vi "ResearcgStandingFrame-V1.1.vi"() -> ()   [LabVIEW 2012]
doc: "Use this template to build a simple state machine design pattern. Each state executes code and determines which state to transition to."
uses:
  controls/State.ctl
panel:
  out "appended array":dbl[](array[numeric])
  out "Scalar":dbl
  out "text":string
  out "substring":string
  in  "Tab Control":T1(tab)
  out "Center Mass Left Force Plate":cluster{dbl[], dbl[]}(graph)={[-7.494780644696312], [-1.1979086821741642]}
  in  "Begin":bool
  in  "stop":bool
  out "Newton Force Readings File Path":path=path "C:/Documents and Settings/z00323/My Documents/Standing Frame/test data/StandingFrameTEST39.dat"
  in  "Newtons":bool
  out "Voltage Readings File Path":path=path "C:/Documents and Settings/z00323/My Documents/Standing Frame/test data/StandingFrameTEST39.dat"
  out "R-FP-Z":dbl
  out "R-FP-Y":dbl
  out "R-FP-X":dbl
  out "R-LC-Z":dbl
  out "R-LC-Y":dbl
  out "R-LC-X":dbl
  out "L-LC-Z":dbl
  out "L-LC-Y":dbl
  out "L-LC-X":dbl
  out "L-FP-X":dbl
  out "L-FP-Y":dbl
  out "L-FP-Z":dbl
  out "String":string caption="Display Unit"
  out "Left Force Plate Z":dbl(slide)=0.43558763460600747 scale=0.0..250.0
  out "Right Force Plate Z":dbl(slide)=0.868584773555102 scale=0.0..250.0
  out "Center Mass Right Force Plate":cluster{dbl[], dbl[]}(graph)
  out "Right Load Cell":cluster{dbl[], dbl[]}(graph)={[0.0, -0.0006862149399022939, 0.0, 0.0], [0.0, 0.005798023167495851, 0.0, 0.0]}
  out "Right Load Cell Z":dbl(slide)=-0.000301685706272135 scale=-50.0..250.0
  out "Left Load Cell Z":dbl(slide)=-0.004073381073294343 scale=-50.0..250.0
  out "Left Load Cell":cluster{dbl[], dbl[]}(graph)={[0.0, -0.0004854170425343219, 0.0, 0.0], [0.0, -0.002818533162237429, 0.0, 0.0]}
  out "Amplitude Unit":string
  out "Right Force PLate Z":dbl(graph)
  out "Left Force Plate Z":dbl(graph)
  out "Right Load Cell Z":dbl(graph)
  out "Right Load Cell Y":dbl(graph)
  out "Right Load Cell X":dbl(graph)
  out "Left Load Cell Z":dbl(graph)
  out "Left Load Cell Y":dbl(graph)
  out "Left Load Cell X":dbl(graph)
  out "Amplitude Unit":string
  in  "Loading- Clibration File Path":path
  in  "Save Calibration Results":bool
  in  "Load Previous Calibration Results":bool
  out "Saving- Clibration File Path":path
  out "Baseline Out":dbl[](array[numeric])
  out "Voltages":dbl[](array[numeric])
  in  "New Calibration":bool
  # "Left Load Cell X\n\nLeft Load Cell Y\n\n\nLeft Load Cell Z\n\nRight Load Cell X\n\n\nRight Load Cell Y\n\nRight Load Cell Z\n\n\nLeft Force Plate X1\n\nLeft Force Plate X2\n\n\nLeft Force Plate Y1\n\nLeft Force PLate Y2\n\n\nLeft Force Plate Z1\n\nLeft Force Plate Z2\n\n\nLeft Force Plate Z3\n\nLeft Force Plate Z4\n\n\nRight Force Plate X1\n\nRight Force Plate X2\n\n\nRight Force Plate Y1\n\nRight Force PLate Y2\n\n\nRight Force Plate Z1\n\nRight Force Plate Z2\n\n\nRight Force Plate Z3\n\nRight Force Plate Z4"
  # "DAQ Board Connections"
  # "LX\nLY\nLZ\nRX\nRY\nRZ\nLFX12\nLFX34\nLFY14\nLFY23\nLFZ1\nLFZ2\nLFZ3\nLFZ4\nRFX12\nRFX34\nRFY14\nRFY23\nRFZ1\nRFZ2\nRFZ3\nRFZ4"
  # "32\n33\n34\n35\n36\n37\n0\n1\n2\n3\n4\n5\n6\n7\n16\n17\n18\n19\n20\n21\n22\n23"
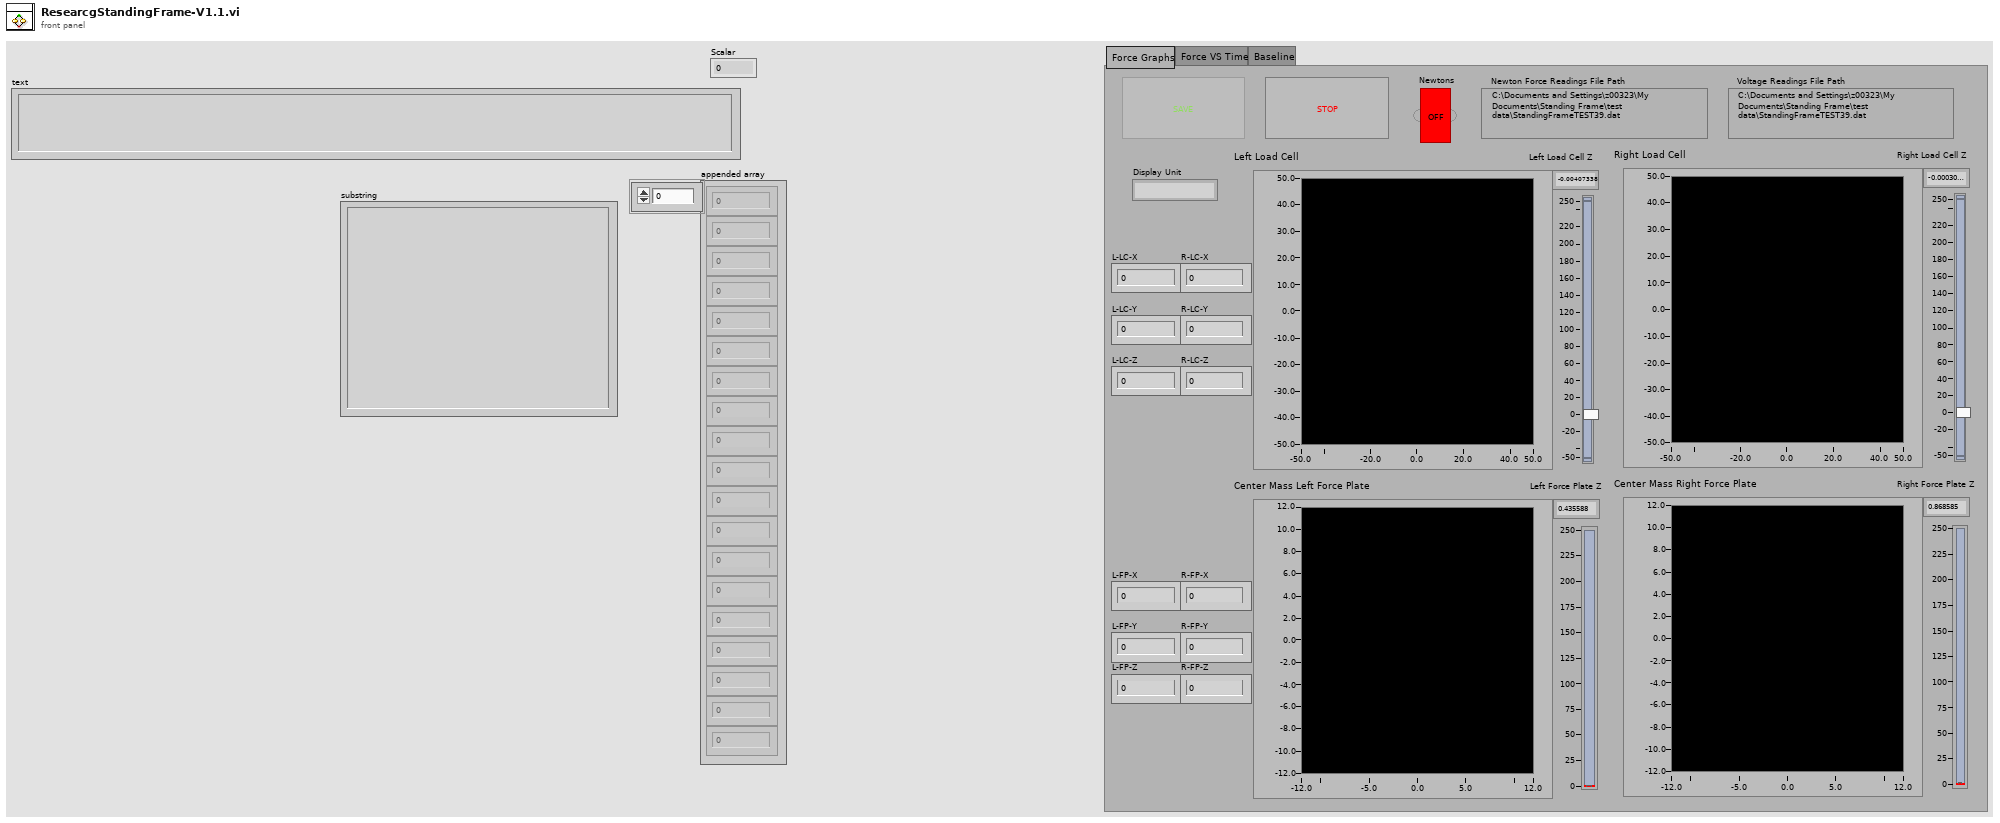
[diagram p1: front panel]
types:
  T1 = enum32{"Force Graphs", "Force VS Time", "Baseline"}
  T2 = typedef "State.ctl" = enum16{"Initialize", "Save", "Main", "Stop"}
  T3 = enum16{"open", "replace", "create", "open or create", "replace or create", "replace or create with confirmation"}
  T4 = enum8{"Enabled", "Disabled", "Disabled and Grayed Out"}
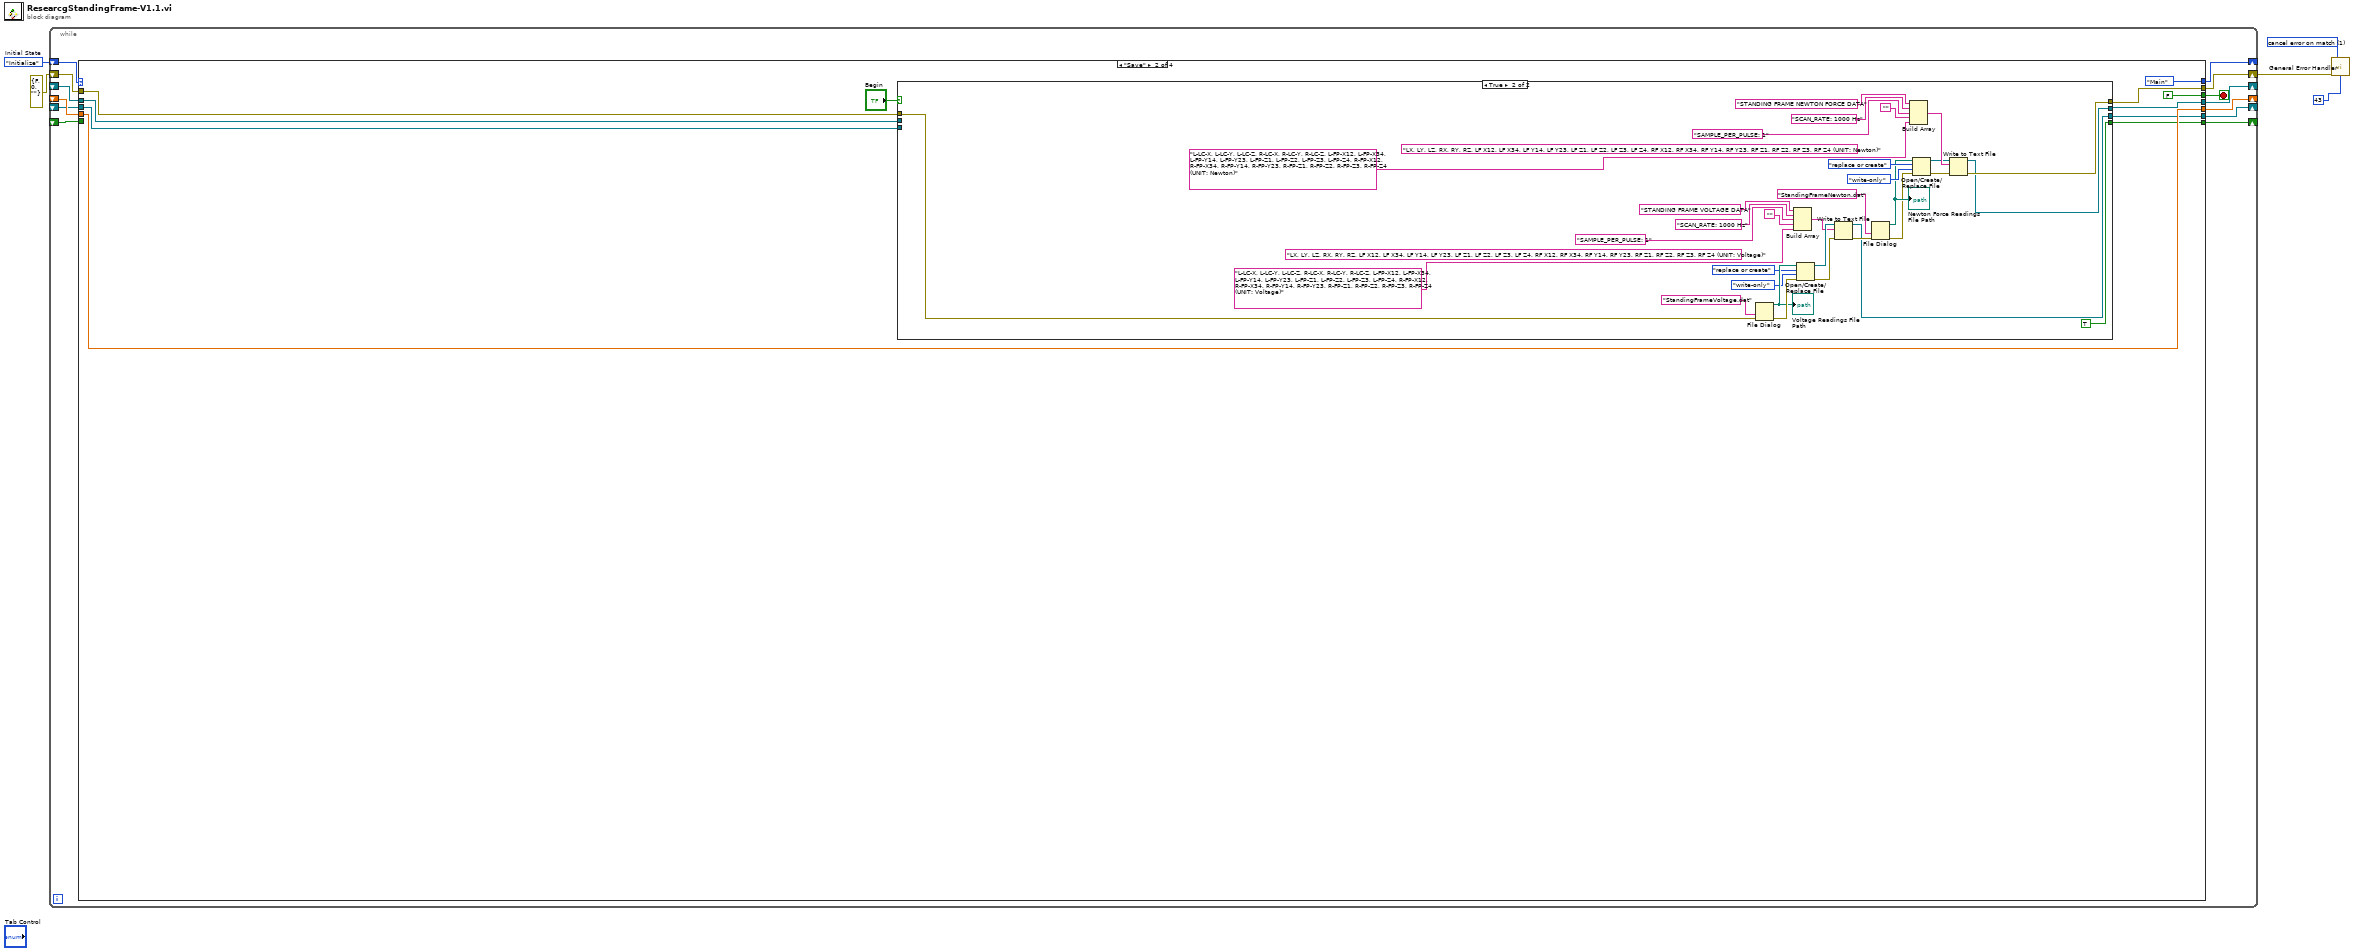
[diagram p0: block diagram]
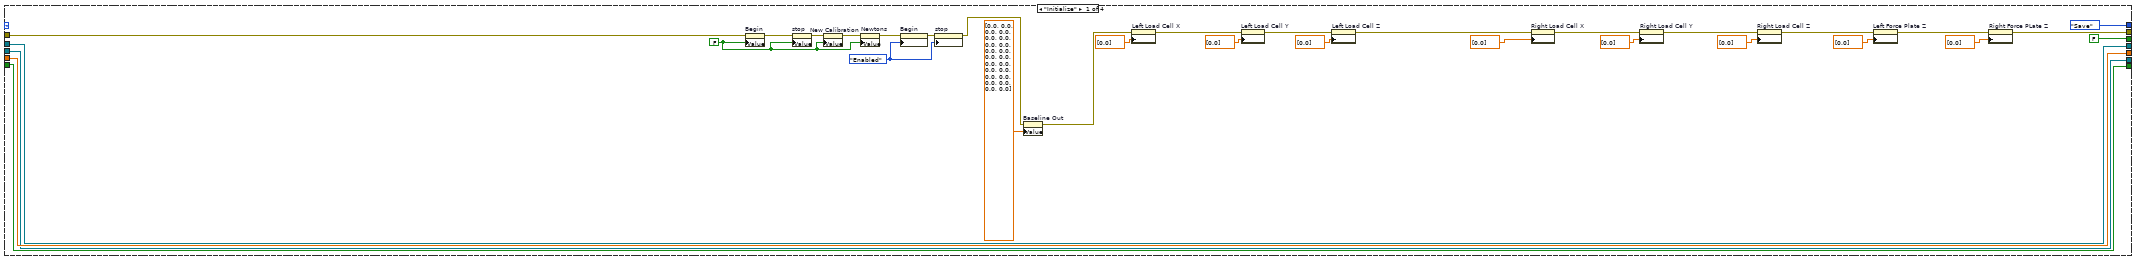
[diagram p2: hidden frame]
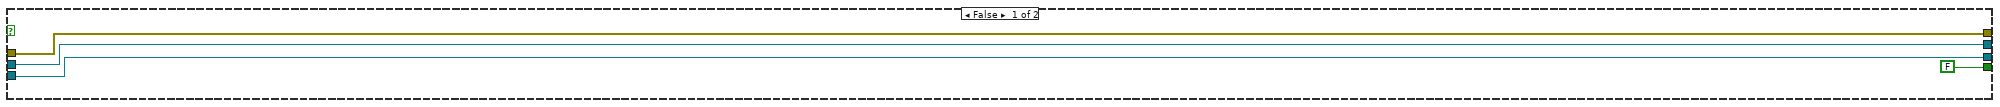
[diagram p3: hidden frame]
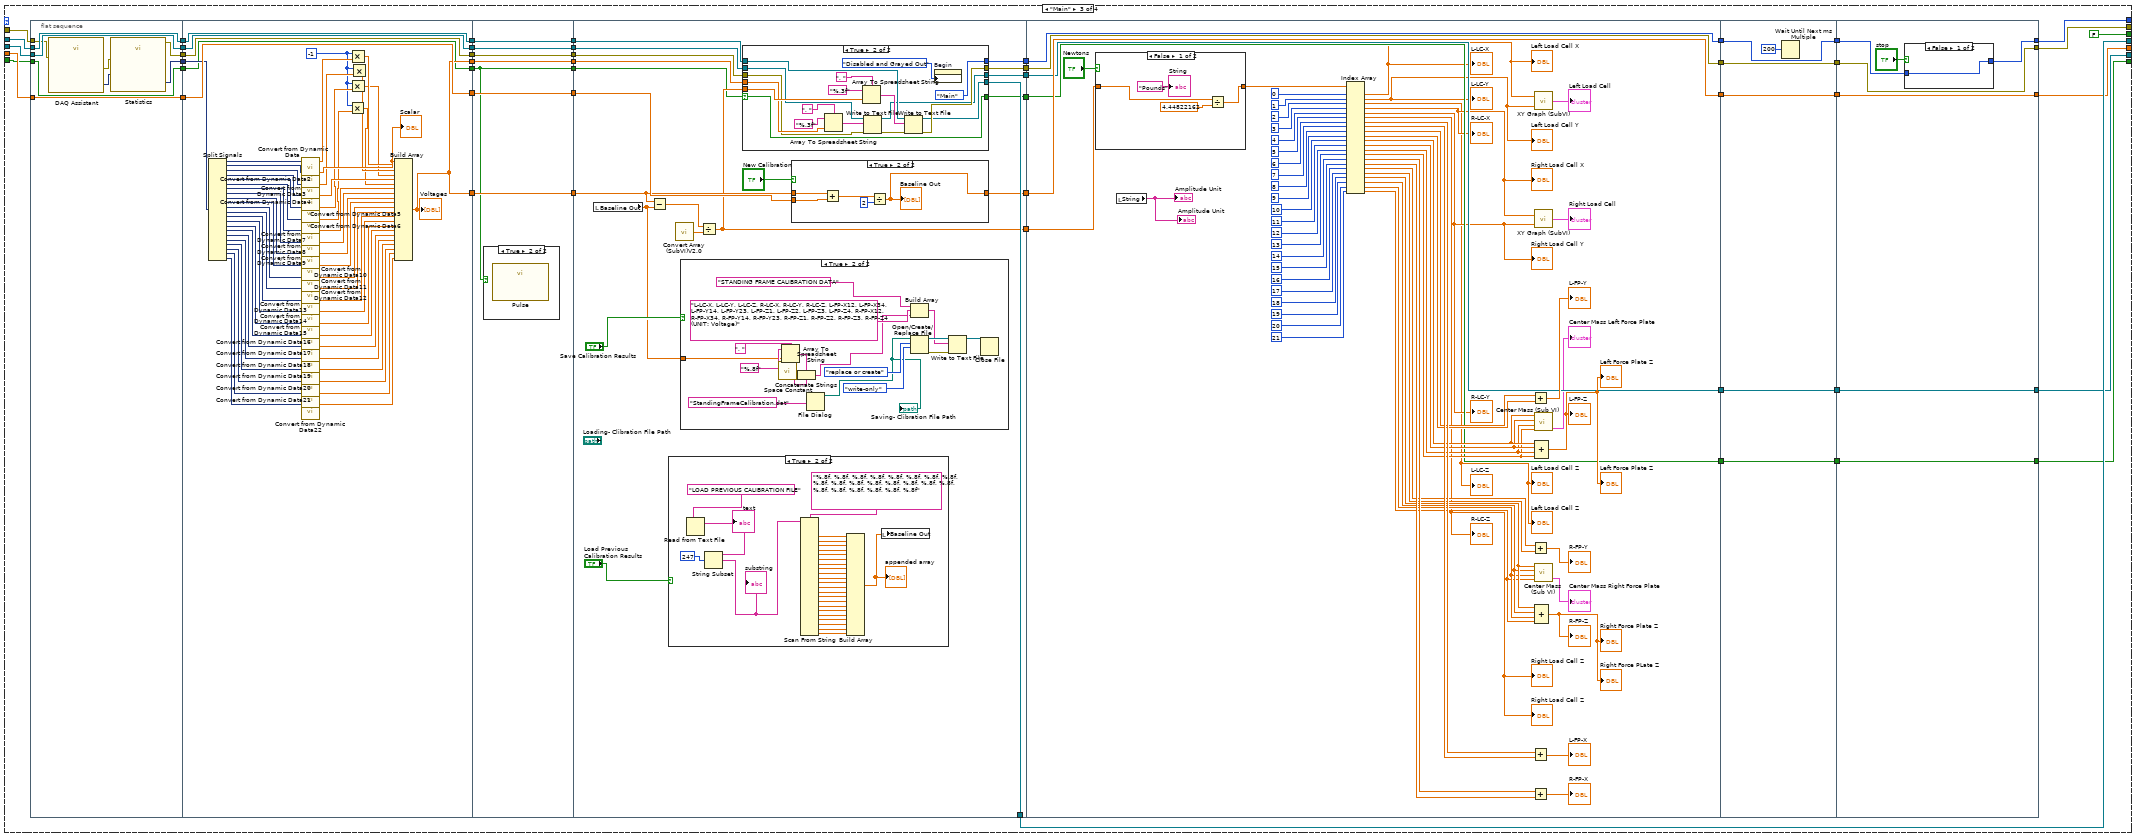
[diagram p4: hidden frame]
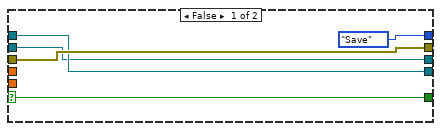
[diagram p8: hidden frame]
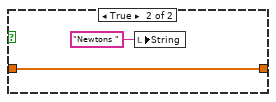
[diagram p10: hidden frame]
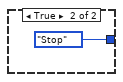
[diagram p11: hidden frame]
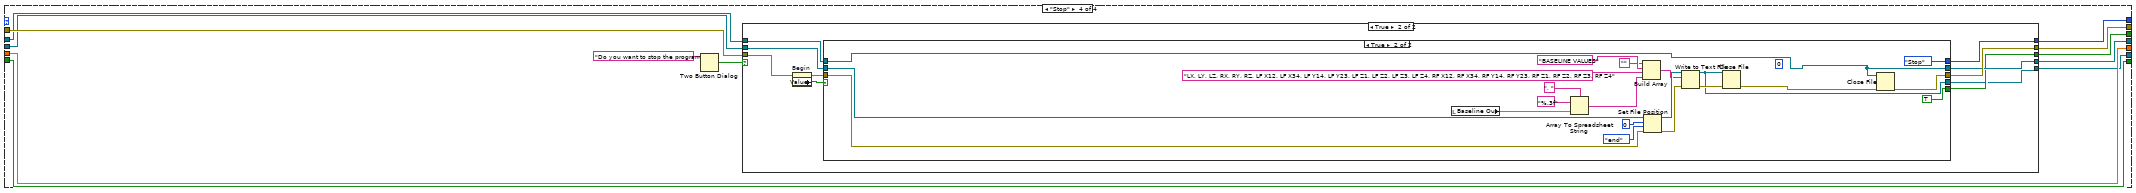
[diagram p12: hidden frame]
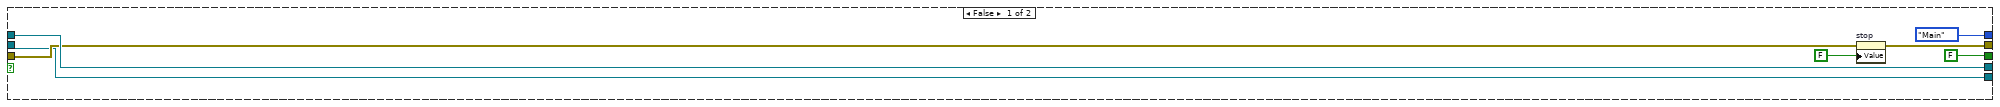
[diagram p13: hidden frame]
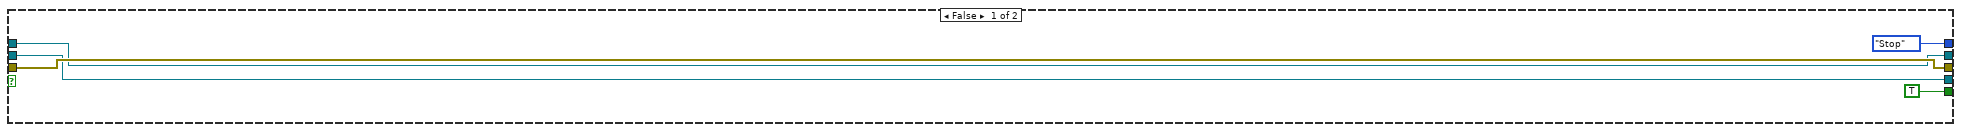
[diagram p14: hidden frame]
diagram:
  w1 = 1 items=["no exception", "cancel error on match", "set error on match"] ("[exception action] (none:0)")
  w5 = State."Initialize"  # Initial State
  n1 = while {
    shift-right: [w17] -> _
    shift-left: w5 -> [w18]
    shift-right: [w12] -> w3
    shift-left: errorcluster {"status"=FALSE, "code"=0, "source"=""} ("error out") -> [w16]
    shift-right: [w14] -> _
    shift-left: _ -> [w13]
    shift-right: [w10] -> _
    shift-left: _ -> [w11]
    shift-right: [w9] -> _
    shift-left: _ -> [w8]
    shift-right: [w7] -> _
    shift-left: _ -> [w6]
    stop <- w15 stop-if-true
    n2 = case shown="\"Save\"" w18 {
      tunnel: [State."Save" ("Next State") State."Main" ("Next State") w144 w405] -> w17
      tunnel: [FALSE ("T button?") FALSE FALSE ("T button?") w404] -> w15
      tunnel: w16 -> [w45 w60 w146 w403]
      tunnel: [w49 w59 w139 w400] -> w14
      tunnel: w13 -> [w49 w56 w145 w401]
      tunnel: [w21 w58 w131 w402] -> w12
      tunnel: w11 -> [w44 w55 w129 w399]
      tunnel: [w44 w55 w125 w399] -> w10
      tunnel: [w41 w52 w124 w398] -> w9
      tunnel: w8 -> [w41 w54 w119 w397]
      tunnel: [w19 w53 w116 w396] -> w7
      tunnel: w6 -> [w19 _ w117 w396]
      frame "Initialize" {
        w38 = FALSE ("Begin")
        w48 = T4."Enabled" ("Disabled")
        n3 = property on="Begin" class="Bool (strict)"(error in=w45, "Value"=w38) -> (error out=w47:errorcluster)  [unwired: 1 in, 1 out]
        n4 = property on="stop" class="Bool (strict)"(error in=w47, "Value"=w38) -> (error out=w43:errorcluster)  [unwired: 1 in, 1 out]
        n5 = property on="New Calibration" class="Bool (strict)"(error in=w43, "Value"=w38) -> (error out=w40:errorcluster)  [unwired: 1 in, 1 out]
        n6 = property on="Newtons" class="Bool (strict)"(error in=w40, "Value"=w38) -> (error out=w39:errorcluster)  [unwired: 1 in, 1 out]
        n7 = property on="Begin" class="Bool (strict)"(error in=w39, "DisabledEnum"=w48) -> (error out=w46:errorcluster)  [unwired: 1 in, 1 out]
        n8 = property on="stop" class="Bool (strict)"(error in=w46, "DisabledEnum"=w48) -> (error out=w20:errorcluster)  [unwired: 1 in, 1 out]
        n9 = property on="Baseline Out" class="Arr (strict)"(error in=w20, "Value"=dbl[] [0.0, 0.0, 0.0, 0.0, 0.0, 0.0, 0.0, 0.0, 0.0, 0.0, 0.0, 0.0, 0.0, 0.0, 0.0, 0.0, 0.0, 0.0, 0.0, 0.0, 0.0, 0.0] ("Baseline Out")) -> (error out=w29:errorcluster)  [unwired: 1 in, 1 out]
        n10 = property on="Left Load Cell X" class="WFChart (strict)"(error in=w29, "History Data"=dbl[] [0.0]) -> (error out=w28:errorcluster)  [unwired: 1 in, 1 out]
        n11 = property on="Left Load Cell Y" class="WFChart (strict)"(error in=w28, "History Data"=dbl[] [0.0]) -> (error out=w27:errorcluster)  [unwired: 1 in, 1 out]
        n12 = property on="Left Load Cell Z" class="WFChart (strict)"(error in=w27, "History Data"=dbl[] [0.0]) -> (error out=w26:errorcluster)  [unwired: 1 in, 1 out]
        n13 = property on="Right Load Cell X" class="WFChart (strict)"(error in=w26, "History Data"=dbl[] [0.0]) -> (error out=w25:errorcluster)  [unwired: 1 in, 1 out]
        n14 = property on="Right Load Cell Y" class="WFChart (strict)"(error in=w25, "History Data"=dbl[] [0.0]) -> (error out=w24:errorcluster)  [unwired: 1 in, 1 out]
        n15 = property on="Right Load Cell Z" class="WFChart (strict)"(error in=w24, "History Data"=dbl[] [0.0]) -> (error out=w23:errorcluster)  [unwired: 1 in, 1 out]
        n16 = property on="Left Force Plate Z" class="WFChart (strict)"(error in=w23, "History Data"=dbl[] [0.0]) -> (error out=w22:errorcluster)  [unwired: 1 in, 1 out]
        n17 = property on="Right Force PLate Z" class="WFChart (strict)"(error in=w22, "History Data"=dbl[] [0.0]) -> (error out=w21:errorcluster)  [unwired: 1 in, 1 out]
      }
      frame "Save" {
        n18 = case shown="True" "Begin" {
          tunnel: w60 -> [w66 w78]
          tunnel: [w65 w92] -> w59
          tunnel: [w66 w94] -> w58
          tunnel: w56 -> [w65 _]
          tunnel: [w64 w76] -> w52
          tunnel: w54 -> [w64 _]
          tunnel: [FALSE TRUE] -> w53
          frame False {
          }
          frame True {
            (unwired) "LX, LY, LZ, RX, RY, RZ, LF X12, LF X34, LF Y14, LF Y23, LF Z1, LF Z2, LF Z3, LF Z4, RF X12, RF X34, RF Y14, RF Y23, RF Z1, RF Z2, RF Z3, RF Z4 (UNIT: Voltage)"
            (unwired) "LX, LY, LZ, RX, RY, RZ, LF X12, LF X34, LF Y14, LF Y23, LF Z1, LF Z2, LF Z3, LF Z4, RF X12, RF X34, RF Y14, RF Y23, RF Z1, RF Z2, RF Z3, RF Z4 (UNIT: Newton)"
            n19 = File Dialog(8:w78, 9:"StandingFrameVoltage.dat" ("default name")) -> (0:w86:errorcluster, 3:w84:path)  [unwired: 1 in, 6 out]
            "Voltage Readings File Path" <- w84
            n20 = Build Array("STANDING FRAME VOLTAGE DATA", "SCAN_RATE: 1000 Hz", "SAMPLE_PER_PULSE: 1", "", "L-LC-X, L-LC-Y, L-LC-Z, R-LC-X, R-LC-Y, R-LC-Z, L-FP-X12, L-FP-X34, L-FP-Y14, L-FP-Y23, L-FP-Z1, L-FP-Z2, L-FP-Z3, L-FP-Z4, R-FP-X12, R-FP-X34, R-FP-Y14, R-FP-Y23, R-FP-Z1, R-FP-Z2, R-FP-Z3, R-FP-Z4 (UNIT: Voltage)") -> (w82:string[])
            n21 = Open/Create/Replace File(file path (use dialog)=w84, error in=w86, operation (0:open)=T3."replace or create", access (0:read/write)=enum16{"read/write", "read-only", "write-only"}."write-only") -> (refnum out=w83:refnum<file>, error out=w87:errorcluster)  [unwired: 3 out]
            n22 = Write to Text File(file (use dialog)=w83, text=w82, error in=w87) -> (refnum out=w76:refnum<file>, error out=w77:errorcluster)  [unwired: 1 in, 1 out]
            n23 = File Dialog(8:w77, 9:"StandingFrameNewton.dat" ("default name")) -> (0:w89:errorcluster, 3:w91:path)  [unwired: 1 in, 6 out]
            "Newton Force Readings File Path" <- w91
            n24 = Build Array("STANDING FRAME NEWTON FORCE DATA", "SCAN_RATE: 1000 Hz", "SAMPLE_PER_PULSE: 1", "", "L-LC-X, L-LC-Y, L-LC-Z, R-LC-X, R-LC-Y, R-LC-Z, L-FP-X12, L-FP-X34, L-FP-Y14, L-FP-Y23, L-FP-Z1, L-FP-Z2, L-FP-Z3, L-FP-Z4, R-FP-X12, R-FP-X34, R-FP-Y14, R-FP-Y23, R-FP-Z1, R-FP-Z2, R-FP-Z3, R-FP-Z4 (UNIT: Newton)") -> (w95:string[])
            n25 = Open/Create/Replace File(file path (use dialog)=w91, error in=w89, operation (0:open)=T3."replace or create", access (0:read/write)=enum16{"read/write", "read-only", "write-only"}."write-only") -> (refnum out=w93:refnum<file>, error out=w88:errorcluster)  [unwired: 3 out]
            n26 = Write to Text File(file (use dialog)=w93, text=w95, error in=w88) -> (refnum out=w92:refnum<file>, error out=w94:errorcluster)  [unwired: 1 in, 1 out]
          }
        }
      }
      frame "Main" {
        n27 = flat-sequence {
          tunnel: w146 -> [w150]
          tunnel: w145 -> [w153]
          tunnel: [w155] -> w142
          tunnel: [w154] -> w141
          tunnel: [w153] -> w140
          tunnel: [w152] -> w130
          tunnel: w129 -> [w152]
          tunnel: [w151] -> w120
          tunnel: w119 -> [w151]
          tunnel: [w149] -> w118
          tunnel: w117 -> [w149]
          tunnel: w142 -> [w187]
          tunnel: [w187] -> w110
          tunnel: w141 -> [w210]
          tunnel: w140 -> [w186]
          tunnel: [w186] -> w112
          tunnel: [w211] -> w108
          tunnel: w130 -> [w211]
          tunnel: [w173] -> w106
          tunnel: [w173] -> w104
          tunnel: [w172] -> w102
          tunnel: w120 -> [w172]
          tunnel: [w167] -> w100
          tunnel: w118 -> [w167]
          tunnel: w112 -> [w218]
          tunnel: [w218] -> w111
          tunnel: w110 -> [w217]
          tunnel: [w217] -> w109
          tunnel: w108 -> [w216]
          tunnel: [w216] -> w107
          tunnel: w106 -> [w215]
          tunnel: [w215] -> w105
          tunnel: w104 -> [w214]
          tunnel: [w214] -> w103
          tunnel: w102 -> [w213]
          tunnel: [w213] -> w101
          tunnel: w100 -> [w212]
          tunnel: [w212] -> w99
          tunnel: [w234] -> w138
          tunnel: [w237] -> w139
          tunnel: w111 -> [w235]
          tunnel: w109 -> [w236]
          tunnel: [w233] -> w137
          tunnel: [w224] -> w136
          tunnel: w107 -> [w232]
          tunnel: w105 -> [w231]
          tunnel: [w230] -> w128
          tunnel: w103 -> [w229]
          tunnel: [w228] -> w121
          tunnel: w101 -> [w227]
          tunnel: w99 -> [w223]
          tunnel: [w222] -> w113
          tunnel: w138 -> [w374]
          tunnel: [w374] -> w135
          tunnel: w137 -> [w321]
          tunnel: w136 -> [w372]
          tunnel: [w321] -> w133
          tunnel: w128 -> [w338]
          tunnel: [w338] -> w127
          tunnel: [w337] -> w122
          tunnel: w121 -> [w337]
          tunnel: [w322] -> w114
          tunnel: w113 -> [w322]
          tunnel: w135 -> [w386]
          tunnel: [w386] -> w134
          tunnel: w133 -> [w384]
          tunnel: [w384] -> w132
          tunnel: w127 -> [w383]
          tunnel: [w383] -> w126
          tunnel: [w382] -> w123
          tunnel: w122 -> [w382]
          tunnel: [w381] -> w115
          tunnel: w114 -> [w381]
          tunnel: [w393] -> w144
          tunnel: w134 -> [w391]
          tunnel: w132 -> [w390]
          tunnel: [w390] -> w131
          tunnel: w126 -> [w389]
          tunnel: [w389] -> w125
          tunnel: [w388] -> w124
          tunnel: w123 -> [w388]
          tunnel: [w387] -> w116
          tunnel: w115 -> [w387]
          frame #0 {
            n28 = call "DAQ Assistant"("error in"=w150) -> ("data"=w147:dynamicdata, "error out"=w148:errorcluster)  [unwired: 16 in, 1 out]
            n29 = call "Statistics"("Signals"=w147, "error in (no error)"=w148) -> ("Arithmetic Mean"=w154:dynamicdata, "error out"=w155:errorcluster)  [unwired: 24 in]
          }
          frame #1 {
            w158 = -1
            n30 = Split Signals(w210) -> (w209:dynamicdata, w208:dynamicdata, w207:dynamicdata, w206:dynamicdata, w205:dynamicdata, w204:dynamicdata, w203:dynamicdata, w202:dynamicdata, w201:dynamicdata, w200:dynamicdata, w199:dynamicdata, w198:dynamicdata, w197:dynamicdata, w196:dynamicdata, w195:dynamicdata, w194:dynamicdata, w193:dynamicdata, w192:dynamicdata, w191:dynamicdata, w190:dynamicdata, w189:dynamicdata, w188:dynamicdata)  [unwired: 22 in]
            n31 = call "Convert from Dynamic Data"("Dynamic Data Type"=w209) -> ("Scalar"=w165:dbl)  [unwired: 3 in]
            n32 = call "Convert from Dynamic Data2"("Dynamic Data Type"=w208) -> ("Scalar"=w166:dbl)  [unwired: 3 in]
            "Scalar" <- w166
            n33 = call "Convert from Dynamic Data3"("Dynamic Data Type"=w207) -> ("Scalar"=w163:dbl)  [unwired: 3 in]
            n34 = call "Convert from Dynamic Data4"("Dynamic Data Type"=w206) -> ("Scalar"=w161:dbl)  [unwired: 3 in]
            n35 = call "Convert from Dynamic Data5"("Dynamic Data Type"=w205) -> ("Scalar"=w160:dbl)  [unwired: 3 in]
            n36 = call "Convert from Dynamic Data6"("Dynamic Data Type"=w204) -> ("Scalar"=w157:dbl)  [unwired: 3 in]
            n37 = call "Convert from Dynamic Data7"("Dynamic Data Type"=w203) -> ("Scalar"=w174:dbl)  [unwired: 3 in]
            n38 = call "Convert from Dynamic Data8"("Dynamic Data Type"=w202) -> ("Scalar"=w175:dbl)  [unwired: 3 in]
            n39 = call "Convert from Dynamic Data9"("Dynamic Data Type"=w201) -> ("Scalar"=w176:dbl)  [unwired: 3 in]
            n40 = call "Convert from Dynamic Data10"("Dynamic Data Type"=w200) -> ("Scalar"=w177:dbl)  [unwired: 3 in]
            n41 = call "Convert from Dynamic Data11"("Dynamic Data Type"=w199) -> ("Scalar"=w171:dbl)  [unwired: 3 in]
            n42 = call "Convert from Dynamic Data12"("Dynamic Data Type"=w198) -> ("Scalar"=w170:dbl)  [unwired: 3 in]
            n43 = call "Convert from Dynamic Data13"("Dynamic Data Type"=w197) -> ("Scalar"=w178:dbl)  [unwired: 3 in]
            n44 = call "Convert from Dynamic Data14"("Dynamic Data Type"=w196) -> ("Scalar"=w169:dbl)  [unwired: 3 in]
            n45 = call "Convert from Dynamic Data15"("Dynamic Data Type"=w195) -> ("Scalar"=w168:dbl)  [unwired: 3 in]
            n46 = call "Convert from Dynamic Data16"("Dynamic Data Type"=w194) -> ("Scalar"=w179:dbl)  [unwired: 3 in]
            n47 = call "Convert from Dynamic Data17"("Dynamic Data Type"=w193) -> ("Scalar"=w180:dbl)  [unwired: 3 in]
            n48 = call "Convert from Dynamic Data18"("Dynamic Data Type"=w192) -> ("Scalar"=w181:dbl)  [unwired: 3 in]
            n49 = call "Convert from Dynamic Data19"("Dynamic Data Type"=w191) -> ("Scalar"=w182:dbl)  [unwired: 3 in]
            n50 = call "Convert from Dynamic Data20"("Dynamic Data Type"=w190) -> ("Scalar"=w183:dbl)  [unwired: 3 in]
            n51 = call "Convert from Dynamic Data21"("Dynamic Data Type"=w189) -> ("Scalar"=w184:dbl)  [unwired: 3 in]
            n52 = call "Convert from Dynamic Data22"("Dynamic Data Type"=w188) -> ("Scalar"=w185:dbl)  [unwired: 3 in]
            n53 = Multiply(x=w158, y=w157) -> (x*y=w156:dbl)
            n54 = Multiply(x=w158, y=w165) -> (x*y=w164:dbl)
            n55 = Multiply(x=w158, y=w160) -> (x*y=w159:dbl)
            n56 = Multiply(x=w158, y=w163) -> (x*y=w162:dbl)
            n57 = Build Array(w166, w164, w162, w159, w161, w156, w174, w175, w176, w177, w171, w170, w178, w169, w168, w179, w180, w181, w182, w183, w184, w185) -> (w173:dbl[])
            "Voltages" <- w173
          }
          frame #2 {
            n58 = case shown="True" w212 {
              frame False {
              }
              frame True {
                n59 = call "Pulse"() -> ()  [unwired: 18 in, 2 out]
              }
            }
          }
          frame #3 {
            n60 = local read "Baseline Out"() -> (w220:dbl[])
            n61 = Subtract(x=w231, y=w220) -> (x-y=w226:dbl[])
            n62 = case shown="True" "Load Previous Calibration Results" {
              frame False {
              }
              frame True {
                n63 = Read from Text File(prompt (Open existing file)="LOAD PREVIOUS CALIBRATION FILE") -> (text=w243:string)  [unwired: 3 in, 3 out]
                "text" <- w243
                n64 = String Subset(string=w243, offset (0)=247) -> (substring=w241:string)  [unwired: 1 in]
                "substring" <- w241
                n65 = Scan From String(format string="%.8f, %.8f, %.8f, %.8f, %.8f, %.8f, %.8f, %.8f, %.8f, %.8f, %.8f, %.8f, %.8f, %.8f, %.8f, %.8f, %.8f, %.8f, %.8f, %.8f, %.8f, %.8f", input string=w241) -> (output 1=w265:dbl, output 2=w264:dbl, output 3=w263:dbl, output 4=w262:dbl, output 5=w261:dbl, output 6=w260:dbl, output 7=w259:dbl, output 8=w258:dbl, output 9=w257:dbl, output 10=w256:dbl, output 11=w255:dbl, output 12=w254:dbl, output 13=w253:dbl, output 14=w252:dbl, output 15=w251:dbl, output 16=w250:dbl, output 17=w249:dbl, output 18=w248:dbl, output 19=w247:dbl, output 20=w246:dbl, output 21=w245:dbl, output 22=w244:dbl)  [unwired: 24 in, 3 out]
                n66 = Build Array(w265, w264, w263, w262, w261, w260, w259, w258, w257, w256, w255, w254, w253, w252, w251, w250, w249, w248, w247, w246, w245, w244) -> (w240:dbl[])
                "appended array" <- w240
                n67 = local write "Baseline Out"(w240) -> ()
              }
            }
            n68 = call "Convert Array  (SubVI)V2.0.vi"() -> ("Conversion Array"=w225:dbl[])  [unwired: 1 in]
            n69 = case shown="True" "Save Calibration Results" {
              tunnel: w220 -> [_ w275]
              frame False {
              }
              frame True {
                n70 = call <vilib>:"Space Constant.vi"() -> ("String"=w270:string)
                n71 = Array To Spreadsheet String(delimiter (Tab)=", ", array=w275, 3:"%.8f") -> (spreadsheet string=w269:string)
                n72 = Concatenate Strings(w270, w269) -> (w268:string)
                n73 = File Dialog(9:"StandingFrameCalibration.dat" ("default name")) -> (3:w267:path)  [unwired: 2 in, 7 out]
                "Saving- Clibration File Path" <- w267
                n74 = Build Array("STANDING FRAME CALIBRATION DATA", "L-LC-X, L-LC-Y, L-LC-Z, R-LC-X, R-LC-Y, R-LC-Z, L-FP-X12, L-FP-X34, L-FP-Y14, L-FP-Y23, L-FP-Z1, L-FP-Z2, L-FP-Z3, L-FP-Z4, R-FP-X12, R-FP-X34, R-FP-Y14, R-FP-Y23, R-FP-Z1, R-FP-Z2, R-FP-Z3, R-FP-Z4 (UNIT: Voltage)", w268) -> (w280:string[])
                n75 = Open/Create/Replace File(file path (use dialog)=w267, operation (0:open)=T3."replace or create", access (0:read/write)=enum16{"read/write", "read-only", "write-only"}."write-only") -> (refnum out=w281:refnum<file>, error out=w282:errorcluster)  [unwired: 1 in, 3 out]
                n76 = Write to Text File(file (use dialog)=w281, text=w280, error in=w282) -> (refnum out=w273:refnum<file>)  [unwired: 1 in, 2 out]
                n77 = Close File(refnum=w273) -> ()  [unwired: 1 in, 2 out]
              }
            }
            n78 = Divide(x=w226, y=w225) -> (x/y=w224:dbl[])
            n79 = case shown="True" w223 {
              selector: w223 -> [w283 w288]
              tunnel: [w287 w302] -> w233
              tunnel: [w285 w301] -> w237
              tunnel: w236 -> [w287 w292]
              tunnel: [State."Save" ("(Value Not Used)") State."Main" ("(Value Not Used)")] -> w234
              tunnel: w235 -> [w285 w298]
              tunnel: w224 -> [_ w299]
              tunnel: w229 -> [_ w293]
              tunnel: [w284 w290] -> w228
              tunnel: w227 -> [w284 w289]
              tunnel: [w283 w288] -> w222
              frame False {
              }
              frame True {
                n80 = Array To Spreadsheet String(delimiter (Tab)=", ", array=w293, 3:"%.3f") -> (spreadsheet string=w294:string)
                n81 = Array To Spreadsheet String(delimiter (Tab)=", ", array=w299, 3:"%.3f") -> (spreadsheet string=w305:string)
                n82 = Write to Text File(file (use dialog)=w289, text=w294, error in=w292) -> (refnum out=w290:refnum<file>, error out=w291:errorcluster)  [unwired: 1 in, 1 out]
                n83 = Write to Text File(file (use dialog)=w298, text=w305, error in=w291) -> (refnum out=w301:refnum<file>, error out=w302:errorcluster)  [unwired: 1 in, 1 out]
                n84 = property on="Begin" class="Bool (strict)"("DisabledEnum"=T4."Disabled and Grayed Out" ("Disabled")) -> ()  [unwired: 2 in, 2 out]
              }
            }
            n85 = case shown="True" "New Calibration" {
              tunnel: w232 -> [_ w307]
              tunnel: w231 -> [w306 w309]
              tunnel: [w306 w308] -> w230
              frame False {
              }
              frame True {
                n86 = Add(x=w309, y=w307) -> (x+y=w311:dbl[])
                n87 = Divide(x=w311, y=2) -> (x/y=w308:dbl[])
                "Baseline Out" <- w308
              }
            }
          }
          frame #4 {
            n88 = case shown="False" "Newtons" {
              tunnel: w372 -> [w377 w379]
              tunnel: [w376 w379] -> w371
              frame False {
                n89 = Divide(x=w377, y=4.44822162) -> (x/y=w376:dbl[])
                "String" <- "Pounds" ("String")
              }
              frame True {
                n90 = local write "String"("Newtons " ("String")) -> ()
              }
            }
            n91 = local read "String"() -> (→"Amplitude Unit" →"Amplitude Unit":string)
            n92 = Index Array(array=w371, index #1=0 ("index (row)"), index #2=1 ("index (row)"), index #3=2 ("index (row)"), index #4=3 ("index (row)"), index #5=4 ("index (row)"), index #6=5 ("index (row)"), index #7=6 ("index (row)"), index #8=7 ("index (row)"), index #9=8 ("index (row)"), index #10=9 ("index (row)"), index #11=10 ("index (row)"), index #12=11 ("index (row)"), index #13=12 ("index (row)"), index #14=13 ("index (row)"), index #15=14 ("index (row)"), index #16=15 ("index (row)"), index #17=16 ("index (row)"), index #18=17 ("index (row)"), index #19=18 ("index (row)"), index #20=19 ("index (row)"), index #21=20 ("index (row)"), index #22=21 ("index (row)")) -> (element #1=w315:dbl, element #2=w316:dbl, element #3=→"L-LC-Z" →"Left Load Cell Z" →"Left Load Cell Z":dbl, element #4=w317:dbl, element #5=w318:dbl, element #6=→"R-LC-Z" →"Right Load Cell Z" →"Right Load Cell Z":dbl, element #7=w348:dbl, element #8=w347:dbl, element #9=w345:dbl, element #10=w344:dbl, element #11=w332:dbl, element #12=w331:dbl, element #13=w330:dbl, element #14=w329:dbl, element #15=w342:dbl, element #16=w341:dbl, element #17=w340:dbl, element #18=w339:dbl, element #19=w328:dbl, element #20=w327:dbl, element #21=w326:dbl, element #22=w325:dbl)
            "L-LC-X" <- w315
            "L-LC-Y" <- w316
            "R-LC-X" <- w317
            "R-LC-Y" <- w318
            "Left Load Cell X" <- w315
            "Left Load Cell Y" <- w316
            "Right Load Cell X" <- w317
            "Right Load Cell Y" <- w318
            n93 = Add(x=w345, y=w344) -> (x+y=→"L-FP-Y":dbl)
            n94 = Add(x=w340, y=w339) -> (x+y=→"R-FP-Y":dbl)
            n95 = Add(x=w348, y=w347) -> (x+y=→"L-FP-X":dbl)
            n96 = Add(x=w342, y=w341) -> (x+y=→"R-FP-X":dbl)
            n97 = call "Center Mass (Sub VI).vi"("Z4"=w329, "Z3"=w330, "Z2"=w331, "Z1"=w332) -> ("XY Graph"=→"Center Mass Left Force Plate":cluster{dbl[], dbl[]})  [unwired: 2 in]
            n98 = call "Center Mass (Sub VI).vi"("Z4"=w325, "Z3"=w326, "Z2"=w327, "Z1"=w328) -> ("XY Graph"=→"Center Mass Right Force Plate":cluster{dbl[], dbl[]})  [unwired: 2 in]
            n99 = call "XY Graph (SubVI).vi"("Y"=w316, "X"=w315) -> ("XY Graph"=→"Left Load Cell":cluster{"array":dbl[], "array":dbl[]})
            n100 = call "XY Graph (SubVI).vi"("Y"=w318, "X"=w317) -> ("XY Graph"=→"Right Load Cell":cluster{"array":dbl[], "array":dbl[]})
            n101 = Compound Arithmetic op=ADD(w332, w331, w330, w329) -> (→"L-FP-Z" →"Left Force Plate Z" →"Left Force Plate Z":dbl)
            n102 = Compound Arithmetic op=ADD(w328, w327, w326, w325) -> (→"R-FP-Z" →"Right Force PLate Z" →"Right Force Plate Z":dbl)
          }
          frame #5 {
            n103 = Wait Until Next ms Multiple(millisecond multiple=u32 200) -> ()  [unwired: 1 out]
          }
          frame #6 {
            n104 = case shown="False" "stop" {
              tunnel: [w394 State."Stop" ("(Value Not Used)")] -> w393
              tunnel: w391 -> [w394 _]
              frame False {
              }
              frame True {
              }
            }
          }
        }
      }
      frame "Stop" {
        n105 = Two Button Dialog(message="Do you want to stop the program?") -> (T button?=w406:bool)  [unwired: 2 in]
        n106 = case shown="True" w406 {
          tunnel: [FALSE w420] -> w404
          tunnel: [State."Main" ("(Value Not Used)") w421] -> w405
          tunnel: w403 -> [w409 w419]
          tunnel: [w410 w424] -> w402
          tunnel: w401 -> [w412 w423]
          tunnel: [w412 w422] -> w400
          tunnel: [w408 w416] -> w398
          tunnel: w397 -> [w408 w415]
          frame False {
            n107 = property on="stop" class="Bool (strict)"(error in=w409, "Value"=FALSE ("stop")) -> (error out=w410:errorcluster)  [unwired: 1 in, 1 out]
          }
          frame True {
            n108 = property on="Begin" class="Bool (strict)"(error in=w419) -> (error out=w418:errorcluster, "Value"=w417:bool)  [unwired: 1 in, 1 out]
            n109 = case shown="True" w417 {
              tunnel: w418 -> [w427 w434]
              tunnel: [w427 w443] -> w424
              tunnel: w423 -> [w426 w432]
              tunnel: [w426 w432] -> w422
              tunnel: [State."Stop" ("(Value Not Used)") State."Stop" ("(Value Not Used)")] -> w421
              tunnel: [TRUE TRUE] -> w420
              tunnel: [w425 w437] -> w416
              tunnel: w415 -> [w425 w436]
              frame False {
              }
              frame True {
                (unwired) 0 ("pos offset (0)")
                n110 = local read "Baseline Out"() -> (w446:dbl[])
                n111 = Array To Spreadsheet String(delimiter (Tab)=", ", array=w446, 3:"%.3f") -> (spreadsheet string=w430:string)
                n112 = Build Array("", "BASELINE VALUES", "LX, LY, LZ, RX, RY, RZ, LF X12, LF X34, LF Y14, LF Y23, LF Z1, LF Z2, LF Z3, LF Z4, RF X12, RF X34, RF Y14, RF Y23, RF Z1, RF Z2, RF Z3, RF Z4", w430) -> (w435:string[])
                n113 = Set File Position(offset (in bytes) (0)=0 ("pos offset (0)"), refnum=w436, from (0:start)=enum16{"start", "end", "current"}."end" ("pos mode (0:2)"), error in=w434) -> (refnum out=w440:refnum<file>, error out=w441:errorcluster)
                n114 = Write to Text File(file (use dialog)=w440, text=w435, error in=w441) -> (refnum out=w437:refnum<file>, error out=w442:errorcluster)  [unwired: 1 in, 1 out]
                n115 = Close File(refnum=w437, error in=w442) -> (error out=w433:errorcluster)  [unwired: 1 out]
                n116 = Close File(refnum=w432, error in=w433) -> (error out=w443:errorcluster)  [unwired: 1 out]
              }
            }
          }
        }
      }
    }
  }
  n117 = call <vilib>:"General Error Handler.vi"("error in (no error)"=w3, "[exception action] (none:0)"=w1, "[exception code]"=43) -> ()  [unwired: 8 in, 5 out]
